vi "setup_furnitures.vi"(8 "error in":errorcluster, 11 "furntures in":refnum<class "Furniture.lvclass">[](array[class])) -> (0 "error out":errorcluster, 1 "setup results":string[](array[string]), 3 "furntures out":refnum<class "Furniture.lvclass">[](array[class]))   [LabVIEW 2021]
uses:
  Furniture/Furniture.lvclass
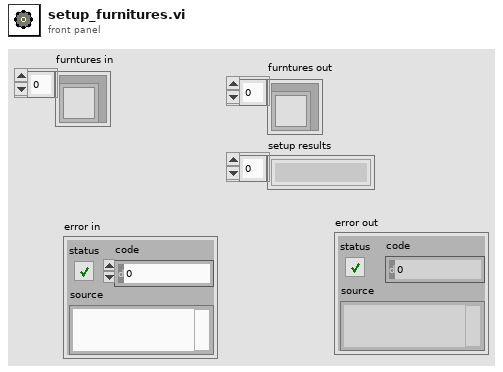
[diagram p1: front panel]
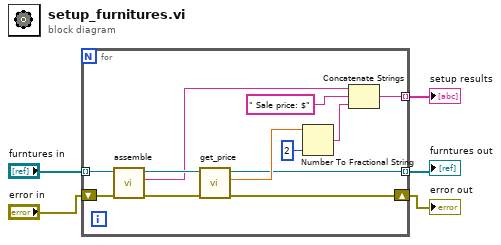
[diagram p0: block diagram]
diagram:
  n1 = for {
    tunnel: "furntures in" -> [w17] mode=indexing
    shift-right: [w13] -> w1
    shift-left: "error in" -> [w15]
    tunnel: [w6] -> w4 mode=indexing
    tunnel: [w7] -> w3 mode=indexing
    n2 = call-dynamic "assemble.vi"("error in (no error)"=w15, "Furniture in"=w17) -> ("error out"=w14:errorcluster, "String"=w12:string, "Furniture out"=w16:refnum<class "Furniture.lvclass">)  [unwired: 7 in]
    n3 = call "get_price.vi"("error in (no error)"=w14, "Furniture in"=w16) -> ("error out"=w13:errorcluster, "price"=w10:dbl, "Furniture out"=w6:refnum<class "Furniture.lvclass">)  [unwired: 7 in]
    n4 = Number To Fractional String(number=w10, precision (6)=i16 2) -> (F-format string=w8:string)  [unwired: 2 in]
    n5 = Concatenate Strings(w12, " Sale price: $" ("string"), w8) -> (w7:string)
  }
  "furntures out" <- w4
  "setup results" <- w3
  "error out" <- w1
